vi "CoordinatePermutations.vi"(7 "Range":dbl=11.0, 8 "NXHP":i32=10, 9 "NXLP":i32=10, 10 "NYHP":i32=10, 11 "NYLP":i32=10) -> (0 "Num Coordinates":i32, 3 "Coordinates":T1(array[cluster]))   [LabVIEW 2014]
uses:
  <vilib>/Analysis/1siggen.llb/Ramp Pattern by Samples.vi
  <vilib>/Analysis/NI_AALBase.lvlib
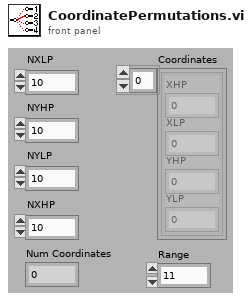
[diagram p1: front panel]
types:
  T1 = cluster{"XHP":i32, "XLP":i32, "YHP":i32, "YLP":i32}[]
  T2 = cluster{"XHP":i32, "XLP":i32, "YHP":i32, "YLP":i32}
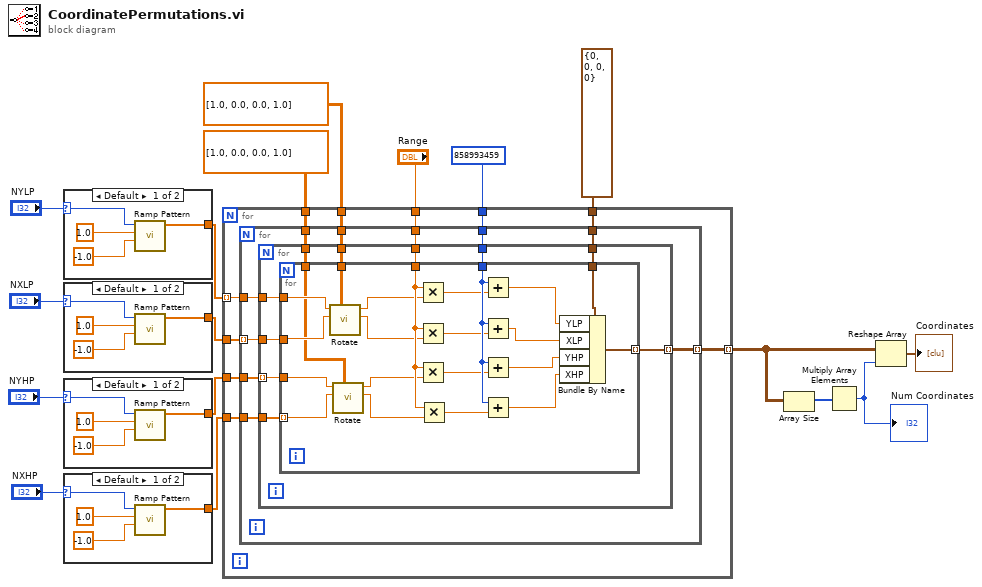
[diagram p0: block diagram]
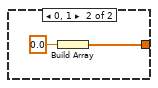
[diagram p2: hidden frame]
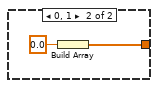
[diagram p3: hidden frame]
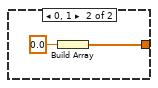
[diagram p4: hidden frame]
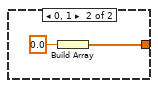
[diagram p5: hidden frame]
diagram:
  n1 = case shown="Default" "NYLP" {
    selector: "NYLP" -> [w18 _]
    tunnel: [w19 w22] -> w5
    frame Default {
      n2 = call-poly <vilib>:"Ramp Pattern.vi"("start"=-1.0, "end"=1.0, "samples"=w18) -> ("Ramp Pattern"=w19:dbl[])  [unwired: 7 in, 1 out]
    }
    frame 0, 1 {
      n3 = Build Array(0.0 ("end")) -> (w22:dbl[])
    }
  }
  n4 = case shown="Default" "NXLP" {
    selector: "NXLP" -> [w24 _]
    tunnel: [w25 w28] -> w7
    frame Default {
      n5 = call-poly <vilib>:"Ramp Pattern.vi"("start"=-1.0, "end"=1.0, "samples"=w24) -> ("Ramp Pattern"=w25:dbl[])  [unwired: 7 in, 1 out]
    }
    frame 0, 1 {
      n6 = Build Array(0.0 ("end")) -> (w28:dbl[])
    }
  }
  n7 = case shown="Default" "NYHP" {
    selector: "NYHP" -> [w30 _]
    tunnel: [w31 w34] -> w8
    frame Default {
      n8 = call-poly <vilib>:"Ramp Pattern.vi"("start"=-1.0, "end"=1.0, "samples"=w30) -> ("Ramp Pattern"=w31:dbl[])  [unwired: 7 in, 1 out]
    }
    frame 0, 1 {
      n9 = Build Array(0.0 ("end")) -> (w34:dbl[])
    }
  }
  n10 = case shown="Default" "NXHP" {
    selector: "NXHP" -> [w36 _]
    tunnel: [w37 w40] -> w17
    frame Default {
      n11 = call-poly <vilib>:"Ramp Pattern.vi"("start"=-1.0, "end"=1.0, "samples"=w36) -> ("Ramp Pattern"=w37:dbl[])  [unwired: 7 in, 1 out]
    }
    frame 0, 1 {
      n12 = Build Array(0.0 ("end")) -> (w40:dbl[])
    }
  }
  n13 = for {
    tunnel: w5 -> [w51] mode=indexing
    tunnel: w7 -> [w50]
    tunnel: w8 -> [w49]
    tunnel: w17 -> [w48]
    tunnel: u32 858993459 ("XHP") -> [w47]
    tunnel: T2 {"XHP"=0, "XLP"=0, "YHP"=0, "YLP"=0} ("Debug.Coordinate") -> [w46]
    tunnel: [w45] -> w12 mode=indexing
    tunnel: "Range" -> [w44]
    tunnel: dbl[][] [[1.0, 0.0], [0.0, 1.0]] -> [w43]
    tunnel: dbl[][] [[1.0, 0.0], [0.0, 1.0]] -> [w42]
    n14 = for {
      tunnel: w51 -> [w61]
      tunnel: w50 -> [w60] mode=indexing
      tunnel: w49 -> [w59]
      tunnel: w48 -> [w58]
      tunnel: w47 -> [w57]
      tunnel: w46 -> [w56]
      tunnel: [w55] -> w45 mode=indexing
      tunnel: w44 -> [w54]
      tunnel: w43 -> [w53]
      tunnel: w42 -> [w52]
      n15 = for {
        tunnel: w61 -> [w71]
        tunnel: w60 -> [w70]
        tunnel: w59 -> [w69] mode=indexing
        tunnel: w58 -> [w68]
        tunnel: w57 -> [w67]
        tunnel: w56 -> [w66]
        tunnel: [w65] -> w55 mode=indexing
        tunnel: w54 -> [w64]
        tunnel: w53 -> [w63]
        tunnel: w52 -> [w62]
        n16 = for {
          tunnel: w71 -> [w81]
          tunnel: w70 -> [w80]
          tunnel: w69 -> [w77]
          tunnel: w68 -> [w76] mode=indexing
          tunnel: w67 -> [w93]
          tunnel: w66 -> [w92]
          tunnel: [w91] -> w65 mode=indexing
          tunnel: w64 -> [w90]
          tunnel: w63 -> [w73]
          tunnel: w62 -> [w72]
          n17 = call "Rotate.vi"("Transform Matrix"=w72, "Y"=w80, "X"=w81) -> ("Yrot"=w79:dbl, "Xrot"=w78:dbl)  [unwired: 6 in, 1 out]
          n18 = call "Rotate.vi"("Transform Matrix"=w73, "Y"=w76, "X"=w77) -> ("Yrot"=w75:dbl, "Xrot"=w74:dbl)  [unwired: 6 in, 1 out]
          n19 = Multiply(x=w90, y=w78) -> (x*y=w89:dbl)
          n20 = Multiply(x=w90, y=w79) -> (x*y=w88:dbl)
          n21 = Multiply(x=w90, y=w74) -> (x*y=w87:dbl)
          n22 = Multiply(x=w90, y=w75) -> (x*y=w86:dbl)
          n23 = Add(x=w93, y=w89) -> (x+y=w85:dbl)
          n24 = Add(x=w93, y=w88) -> (x+y=w82:dbl)
          n25 = Add(x=w93, y=w87) -> (x+y=w83:dbl)
          n26 = Add(x=w93, y=w86) -> (x+y=w84:dbl)
          n27 = Bundle By Name(cluster=w92, "YLP"=w85, "XLP"=w82, "YHP"=w83, "XHP"=w84) -> (w91:T2)
        }
      }
    }
  }
  n28 = Array Size(array=w12) -> (size(s)=w13:i32[])
  n29 = Multiply Array Elements(1:w13) -> (0:w11:i32)
  "Num Coordinates" <- w11
  n30 = Reshape Array(w12, w11) -> (→"Coordinates":T1)
